vi "Worktable.vi"() -> ()   [LabVIEW 2011]
panel:
  in  "Work Table":T1
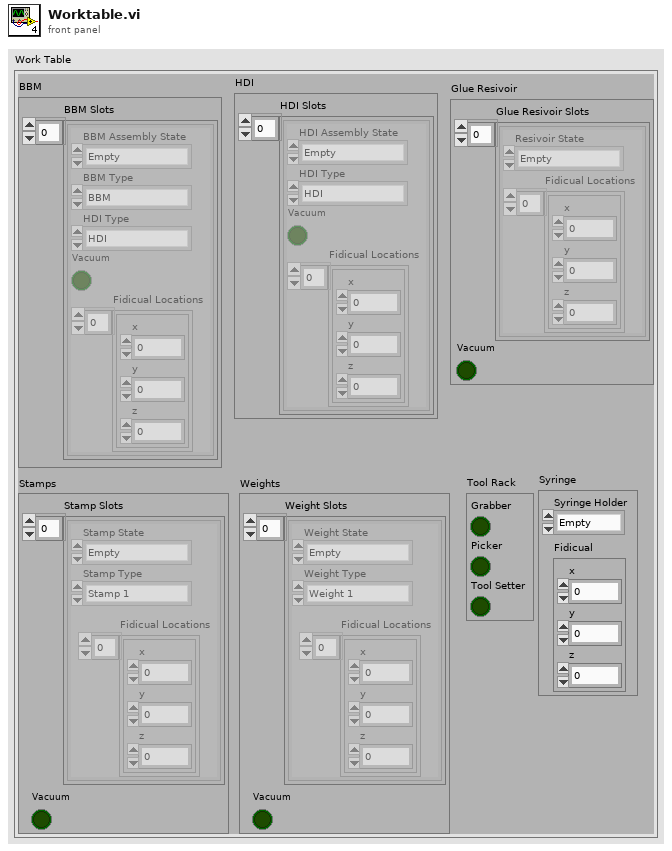
[diagram p1: front panel]
types:
  T1 = cluster{"BBM":cluster{"BBM Slots":cluster{"BBM Assembly State":enum16{"Empty", "Unglued", "Stamped", "PartOnTop", "Weighted"}, "BBM Type":enum16{"BBM", "GlassSlide"}, "HDI Type":enum16{"HDI", "Polyimide"}, "Vacuum":bool, "Fidicual Locations":cluster{"x":dbl, "y":dbl, "z":dbl}[]}[]}, "HDI":cluster{"HDI Slots":cluster{"HDI Assembly State":enum16{"Empty", "Populated"}, "HDI Type":enum16{"HDI", "Polyimide"}, "Vacuum":bool, "Fidicual Locations":cluster{"x":dbl, "y":dbl, "z":dbl}[]}[]}, "Glue Resivoir":cluster{"Glue Resivoir Slots":cluster{"Resivoir State":enum16{"Empty", "Full", "Used"}, "Fidicual Locations":cluster{"x":dbl, "y":dbl, "z":dbl}[]}[], "Vacuum":bool}, "Stamps":cluster{"Stamp Slots":cluster{"Stamp State":enum16{"Empty", "Populated", "Used"}, "Stamp Type":enum16{"Stamp 1", "Stamp 2", "Stamp 3", "Stamp 4"}, "Fidicual Locations":cluster{"x":dbl, "y":dbl, "z":dbl}[]}[], "Vacuum":bool}, "Weights":cluster{"Weight Slots":cluster{"Weight State":enum16{"Empty", "Populated"}, "Weight Type":enum16{"Weight 1", "Weight 2", "Weight 3", "Weight 4"}, "Fidicual Locations":cluster{"x":dbl, "y":dbl, "z":dbl}[]}[], "Vacuum":bool}, "Tool Rack":cluster{"Grabber":bool, "Picker":bool, "Tool Setter":bool}, "Syringe":cluster{"Syringe Holder":enum16{"Empty", "Populated", "Calibrated"}, "Fidicual ":cluster{"x":dbl, "y":dbl, "z":dbl}}}
  T2 = cluster{"BBM Slots":cluster{"BBM Assembly State":enum16{"Empty", "Unglued", "Stamped", "PartOnTop", "Weighted"}, "BBM Type":enum16{"BBM", "GlassSlide"}, "HDI Type":enum16{"HDI", "Polyimide"}, "Vacuum":bool, "Fidicual Locations":cluster{"x":dbl, "y":dbl, "z":dbl}[]}[]}
  T3 = cluster{"HDI Slots":cluster{"HDI Assembly State":enum16{"Empty", "Populated"}, "HDI Type":enum16{"HDI", "Polyimide"}, "Vacuum":bool, "Fidicual Locations":cluster{"x":dbl, "y":dbl, "z":dbl}[]}[]}
  T4 = cluster{"BBM Assembly State":enum16{"Empty", "Unglued", "Stamped", "PartOnTop", "Weighted"}, "BBM Type":enum16{"BBM", "GlassSlide"}, "HDI Type":enum16{"HDI", "Polyimide"}, "Vacuum":bool, "Fidicual Locations":cluster{"x":dbl, "y":dbl, "z":dbl}[]}[]
  T5 = enum16{"Empty", "Unglued", "Stamped", "PartOnTop", "Weighted"}
  T6 = cluster{"BBM Assembly State":enum16{"Empty", "Unglued", "Stamped", "PartOnTop", "Weighted"}, "BBM Type":enum16{"BBM", "GlassSlide"}, "HDI Type":enum16{"HDI", "Polyimide"}, "Vacuum":bool, "Fidicual Locations":cluster{"x":dbl, "y":dbl, "z":dbl}[]}
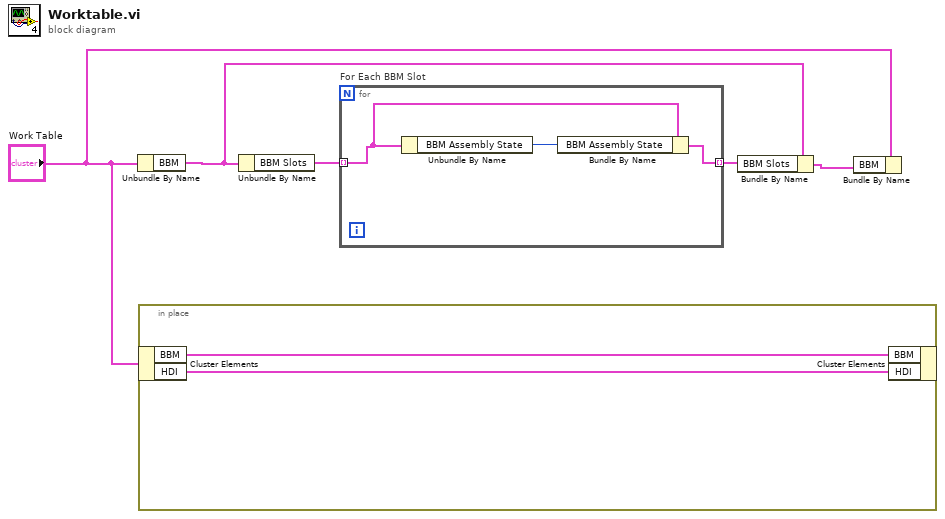
[diagram p0: block diagram]
diagram:
  n1 = Unbundle By Name("Work Table") -> ("BBM"=w4:T2)
  n2 = in-place {
    n3 = in-place-cluster #1("Work Table") -> ("BBM"=w7:T2, "HDI"=w6:T3)
    n4 = in-place-cluster #1("BBM"=w7, "HDI"=w6) -> ()  [unwired: 1 out]
  }
  n5 = Unbundle By Name(w4) -> ("BBM Slots"=w5:T4)
  n6 = for "For Each BBM Slot" {
    tunnel: w5 -> [w8] mode=indexing
    tunnel: [w9] -> w2 mode=indexing
    n7 = Unbundle By Name(w8) -> ("BBM Assembly State"=w10:T5)
    n8 = Bundle By Name(cluster=w8, "BBM Assembly State"=w10) -> (w9:T6)
  }
  n9 = Bundle By Name(cluster=w4, "BBM Slots"=w2) -> (w3:T2)
  n10 = Bundle By Name(cluster="Work Table", "BBM"=w3) -> ()  [unwired: 1 out]
